vi "NML Data Acquisition-old.vi"() -> ()   [LabVIEW 2019]
doc: "This VI is designed to scan data each time the the trigger channel changes by an amount ∆ trigger. The first data column is converted to tesla using the magnet ID (or 'None' for volts).\nScott Hannahs, NHMFL - FSU, Mar 1996"
panel:
  in  "Configure":bool
  in  "Show help":bool
  in  "Display?":bool[](array[boolean])=[FALSE, FALSE, FALSE, FALSE, FALSE, FALSE, FALSE, FALSE, FALSE, FALSE, FALSE, FALSE, FALSE, FALSE, FALSE]
  out "# of columns":i32
  out "Index":i32
  out "Data Array":dbl[][](array[numeric]) format="%.2f"
  in  "Print":bool
  out "Data Record":string
  in  "Column Headings":string[](array[string])=["Field", "Voltage1", "Voltage2", "Temp", "Timestamp", "", "", "", "", "", "", "", "", "", ""]
  in  "Scale Factors":dbl[](array[numeric])=[1.0, 1.0, 1.0, 1.0, 1.0, 1.0, 1.0, 1.0, 1.0, 1.0, 1.0, 1.0, 1.0, 1.0, 1.0, 1.0, 1.0, 1.0, 1.0] format="%.3e"
  in  "Magnet ID":i32(ring) items=["None"]
  in  "Comments":string="This data's for you!\n"
  in  "Monopolar\n\n\n\nBipolar":bool
  in  "Points Averaged":i32=128 min=1 max=32000 step=1
  out "Mode Indicator":string="Standby"
  in  "User Name":string="Conan The Scientist"
  in  "File Name":string="Test"
  in  "TEST\nGPIB":bool
  in  "New/Stop":bool
  in  "X-Axis":i32(ring)=1 items=["Point #", "Field", "Voltage1", "Voltage2", "Temp", "Timestamp", "", "", "", "", "", "", "", "", "", ""]
  in  "Pause":bool=TRUE
  out "Data Plot":cluster{dbl[], dbl[]}[](graph)
  in  "CHANNEL & RANGE SELECTOR":T1 {"0" scale=0.0..4.0; "7" scale=0.0..4.0; "6" scale=0.0..4.0; "5" scale=0.0..4.0; "4" scale=0.0..4.0; "3" scale=0.0..4.0; "2" scale=0.0..4.0; "1" scale=0.0..4.0}
  in  "Æ Trigger":dbl=0.025 min=0.0 format="%.3f"
  in  "Trigger Column":i32(ring)=1 items=["Time", "Field", "Voltage1", "Voltage2", "Temp", "Timestamp", "", "", "", "", "", "", "", "", "", ""]
  # "Run"
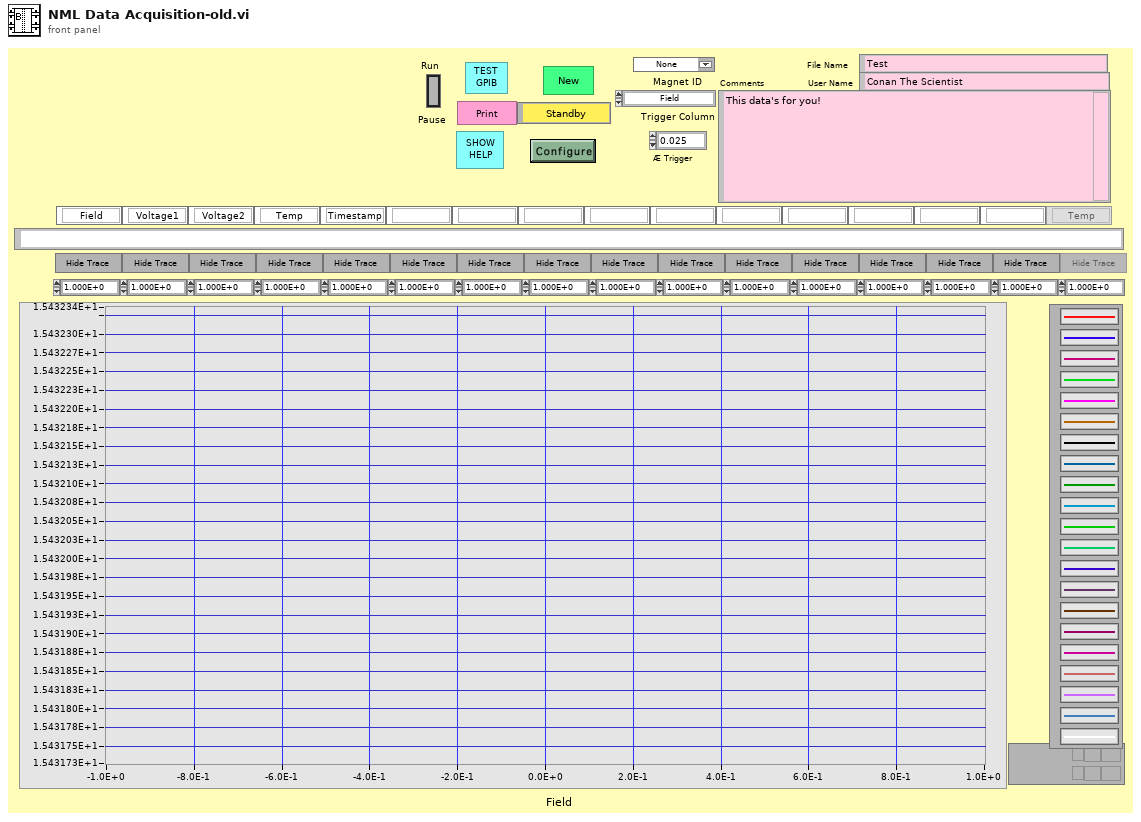
[diagram p1: front panel]
types:
  T1 = cluster{"0":i16, "1":i16, "2":i16, "3":i16, "4":i16, "5":i16, "6":i16, "7":i16}
  T2 = cluster{"Current Scale Factor kA/V":dbl, "I->B":dbl[], "B->I":dbl[]}
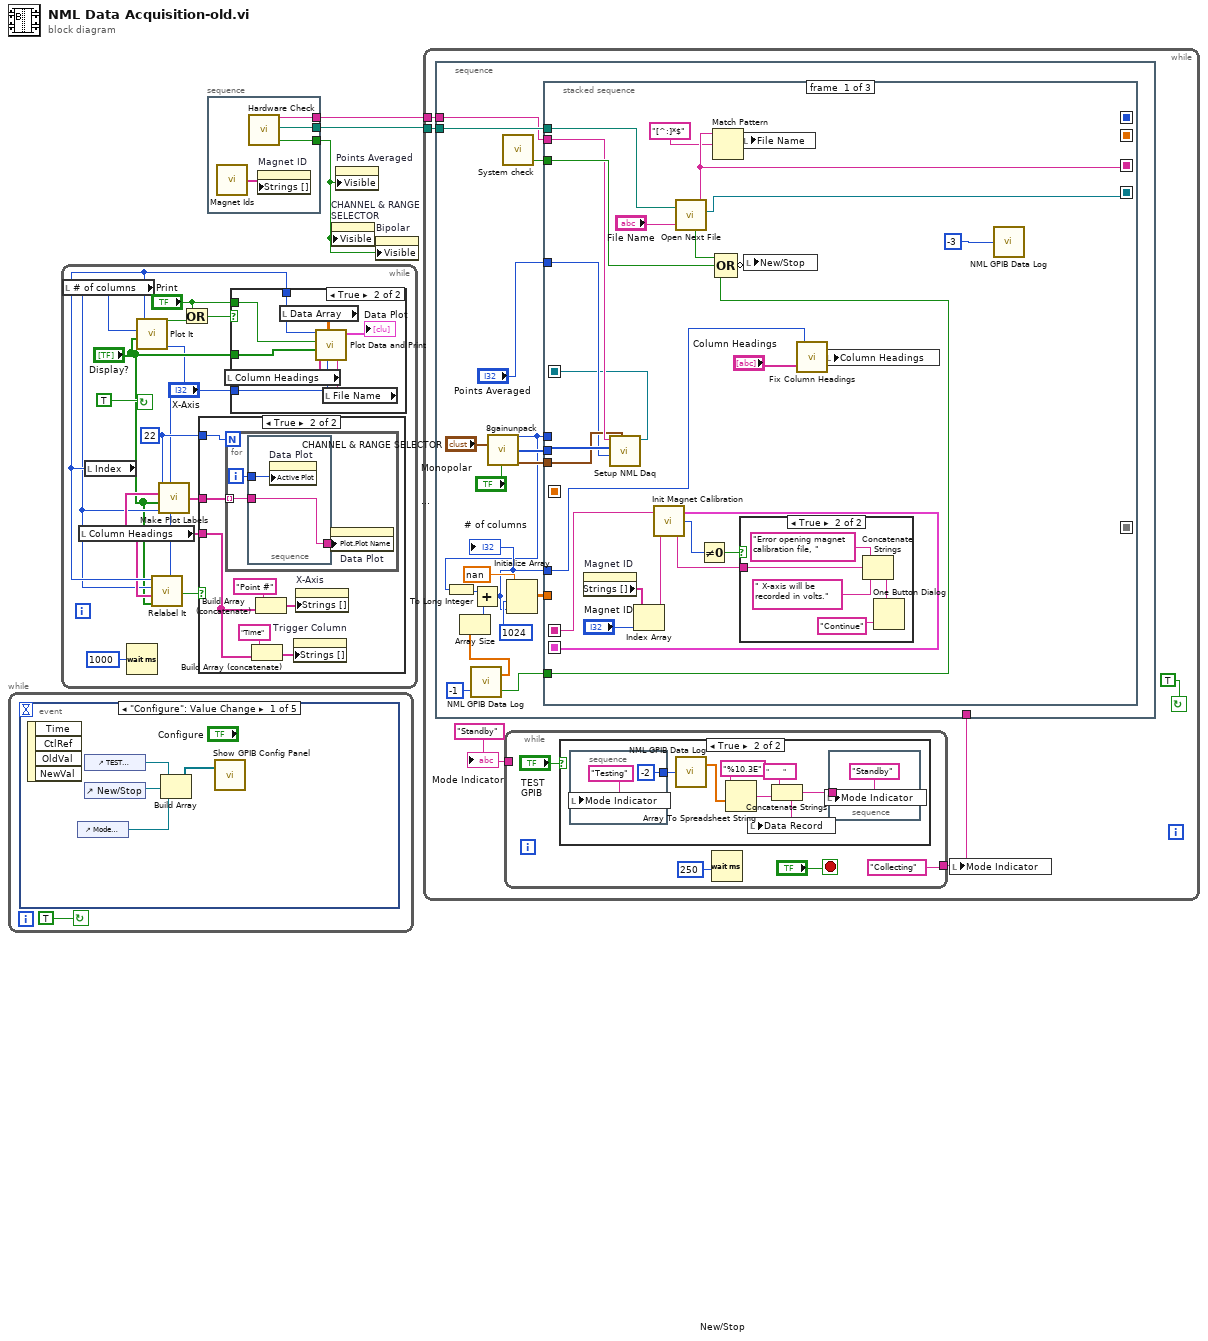
[diagram p0: block diagram]
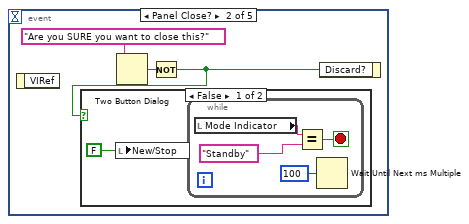
[diagram p2: hidden frame]
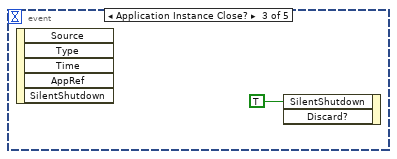
[diagram p4: hidden frame]
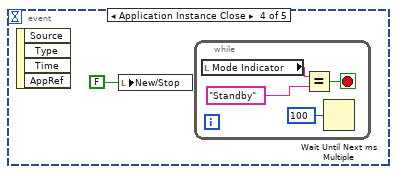
[diagram p5: hidden frame]
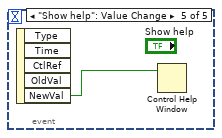
[diagram p6: hidden frame]
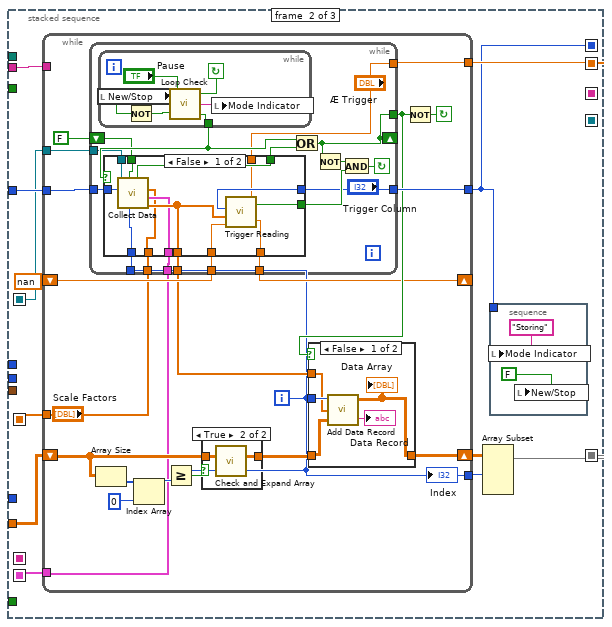
[diagram p9: hidden frame]
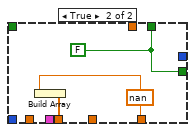
[diagram p10: hidden frame]
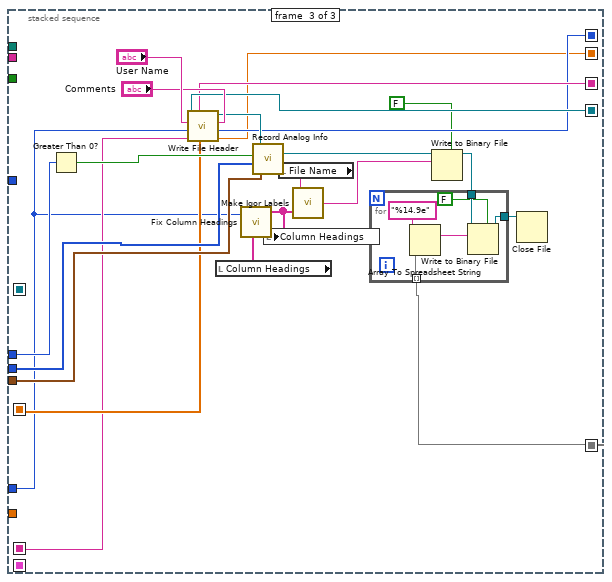
[diagram p13: hidden frame]
diagram:
  n1 = while {
    stop <- TRUE continue-if-true
    n2 = event shown="[0] \"Configure\": Value Change" {
      selector: _ -> [_ _ _ _ _]
      dyn-events: _ -> [_ _ _ _ _]
      timeout: _ -> [_ _ _ _ _]
      event "Configure": Value Change {
        n3 = event-data() -> ()  [unwired: 1 in, 4 out]
        n4 = control-ref of="Mode Indicator"() -> (w5:refnum<vi>)
        n5 = control-ref of="TEST\nGPIB"() -> (w7:refnum<vi>)
        n6 = control-ref of="New/Stop"() -> (w6:refnum<vi>)
        n7 = Build Array(w7, w6, w5) -> (w8:refnum<vi>[])
        n8 = call "Show GPIB Config Panel.vi"("Array"=w8) -> ()  [unwired: 1 in, 1 out]
      }
      event Panel Close? {
        n9 = event-data() -> ()  [unwired: 1 in, 1 out]
        n10 = Two Button Dialog(message="Are you SURE you want to close this?") -> (T button?=w10:bool)  [unwired: 2 in]
        n11 = Not(x=w10) -> (.not. x?=w9:bool)
        n12 = case shown="False" w9 {
          frame False {
            n13 = local write "New/Stop"(FALSE ("New/Stop")) -> ()
            n14 = while {
              stop <- w15 stop-if-true
              n15 = local read "Mode Indicator"() -> (w16:string)
              n16 = Equal?(x=w16, y="Standby") -> (x = y?=w15:bool)
              n17 = Wait Until Next ms Multiple(millisecond multiple=u32 100) -> ()  [unwired: 1 out]
            }
          }
          frame True {
          }
        }
        n18 = event-data("Discard?"=w9) -> ()  [unwired: 1 in, 1 out]
      }
      event Application Instance Close? {
        n19 = event-data() -> ()  [unwired: 1 in, 5 out]
        n20 = event-data("SilentShutdown"=TRUE) -> ()  [unwired: 2 in, 1 out]
      }
      event Application Instance Close {
        n21 = event-data() -> ()  [unwired: 1 in, 4 out]
        n22 = local write "New/Stop"(FALSE ("New/Stop")) -> ()
        n23 = while {
          stop <- w21 stop-if-true
          n24 = local read "Mode Indicator"() -> (w22:string)
          n25 = Equal?(x=w22, y="Standby") -> (x = y?=w21:bool)
          n26 = Wait Until Next ms Multiple(millisecond multiple=u32 100) -> ()  [unwired: 1 out]
        }
      }
      event "Show help": Value Change {
        n27 = event-data() -> ("NewVal"=w23:bool)  [unwired: 1 in, 4 out]
        n28 = Control Help Window(1:w23) -> ()  [unwired: 1 in]
      }
    }
  }
  n29 = while {
    stop <- TRUE continue-if-true
    w28 = 22
    n30 = local read "# of columns"() -> (w26:i32)
    n31 = local read "Column Headings"() -> (w27:string[])
    n32 = local read "Index"() -> (w30:i32)
    n33 = Wait (ms)(milliseconds to wait=u32 1000) -> ()  [unwired: 1 out]
    n34 = call "Plot It.vi"("X-Axis"="X-Axis", "Display?"="Display?", "# of columns"=w26, "Index"=w30) -> (0:w32:bool)
    n35 = call "Relabel It.vi"("Index"=w30, "# of columns"=w26, "Column Headings"=w27, "Display?"="Display?", "X-Axis"="X-Axis") -> (5:w34:bool)
    n36 = call "Make Plot Labels.vi"("Plot Size"=w28, "Column Headings"=w27, "Display?"="Display?", "# of columns"=w26, "X-axis"="X-Axis") -> ("Plot Names"=w29:string[])
    n37 = Or(x="Print", y=w32) -> (x .or. y?=w33:bool)
    n38 = case shown="True" w34 {
      tunnel: w27 -> [_ w37]
      tunnel: w28 -> [_ w39]
      tunnel: w29 -> [_ w38]
      frame False {
      }
      frame True {
        n39 = for {
          N: w39 -> [_]
          tunnel: w38 -> [w44] mode=indexing
          i -> [w46]
          n40 = stacked-sequence {
            tunnel: w46 -> [w48]
            tunnel: [w47] -> w45
            tunnel: w44 -> [w47]
            frame #0 {
              n41 = property on="Data Plot" class="XYGraph (strict)"("Active Plot"=w48) -> ()  [unwired: 2 in, 2 out]
            }
          }
          n42 = property on="Data Plot" class="XYGraph (strict)"("Plot.Plot Name"=w45) -> ()  [unwired: 2 in, 2 out]
        }
        n43 = Build Array (concatenate)("Time", w37) -> (w43:string[])
        n44 = Build Array (concatenate)("Point #", w37) -> (w41:string[])
        n45 = property on="Trigger Column" class="Ring (strict)"("Strings []"=w43) -> ()  [unwired: 2 in, 2 out]
        n46 = property on="X-Axis" class="Ring (strict)"("Strings []"=w41) -> ()  [unwired: 2 in, 2 out]
      }
    }
    n47 = case shown="True" w33 {
      tunnel: "Display?" -> [_ w56]
      tunnel: w30 -> [_ w55]
      tunnel: "X-Axis" -> [_ w50]
      tunnel: "Print" -> [_ w49]
      frame False {
      }
      frame True {
        n48 = local read "Column Headings"() -> (w51:string[])
        n49 = local read "Data Array"() -> (w52:dbl[][])
        n50 = local read "File Name"() -> (w54:string)
        n51 = call "Plot Data and Print.vi"("File:"=w54, "x axis column"=w50, "Data"=w52, "Col heading"=w51, "Display/hide"=w56, "Print"=w49, "Index"=w55) -> ("Data Plot"=→"Data Plot":cluster{dbl[], dbl[]}[])  [unwired: 2 in]
      }
    }
  }
  n52 = stacked-sequence {
    tunnel: [w59] -> w1
    tunnel: [w58] -> w2
    tunnel: [w57] -> w3
    frame #0 {
      n53 = call "Magnet Ids.vi"() -> ("Magnet IDs"=w60:string[])
      n54 = call "Hardware Check.vi"() -> ("Data Acq Device"=w57:string, "Data Directory Path"=w59:path, "Has A/D board"=w58:bool)  [unwired: 1 in]
      n55 = property on="Magnet ID" class="Ring (strict)"("Strings []"=w60) -> ()  [unwired: 2 in, 2 out]
    }
  }
  n56 = property on="CHANNEL & RANGE SELECTOR" class="Clust (strict)"("Visible"=w2) -> ()  [unwired: 2 in, 2 out]
  n57 = property on="Points Averaged" class="DigNum (strict)"("Visible"=w2) -> ()  [unwired: 2 in, 2 out]
  n58 = property on="Bipolar" class="Bool (strict)"("Visible"=w2) -> ()  [unwired: 2 in, 2 out]
  n59 = while {
    tunnel: w3 -> [w63]
    tunnel: w1 -> [w64]
    stop <- TRUE continue-if-true
    w62 = "Standby"
    n60 = while {
      tunnel: ["Collecting"] -> w61
      tunnel: w62 -> [_]
      stop <- "New/Stop" stop-if-true
      n61 = case shown="True" "TEST\nGPIB" {
        frame False {
        }
        frame True {
          n62 = stacked-sequence {
            tunnel: [-2] -> w71
            frame #0 {
              n63 = local write "Mode Indicator"("Testing") -> ()
            }
          }
          n64 = call "NML GPIB Data Log.vi"("Point #"=w71) -> ("GPIB Data"=w70:dbl[])  [unwired: 1 out]
          n65 = Array To Spreadsheet String(array=w70, 3:"%10.3E") -> (spreadsheet string=w73:string)  [unwired: 1 in]
          n66 = Concatenate Strings("       ", w73) -> (w74:string)
          n67 = local write "Data Record"(w74) -> ()
          n68 = stacked-sequence {
            tunnel: w74 -> [_]
            frame #0 {
              n69 = local write "Mode Indicator"("Standby") -> ()
            }
          }
        }
      }
      n70 = Wait (ms)(milliseconds to wait=u32 250) -> ()  [unwired: 1 out]
    }
    n71 = stacked-sequence {
      tunnel: w64 -> [w89]
      tunnel: w63 -> [w88]
      tunnel: w61 -> [_]
      frame #0 {
        n72 = call "NML GPIB Data Log.vi"("Point #"=-1) -> ("GPIB Data"=w80:dbl[], "Stop"=w81:bool)
        n73 = Array Size(array=w80) -> (size(s)=w94:i32)
        n74 = call "8gainunpack.vi"("GAIN & CHANNEL SELECTOR"="CHANNEL & RANGE SELECTOR", "Monopolar"="Monopolar\n\n\n\nBipolar") -> ("Number of channels"=w82:i32, "channels (0)"=w93:i32[], "Input Limits"=w96:cluster{"High Limit":dbl, "Low Limit":dbl}[])
        n75 = To Long Integer(number=w82) -> (32bit integer=w95:i32)
        n76 = Add(x=w95, y=w94) -> (x+y=w85:i32)
        "# of columns" <- w85
        n77 = call "System check.vi"() -> ("Abort"=w84:bool)  [unwired: 3 in]
        n78 = Initialize Array(nan, 1024, w85) -> (w92:dbl[][])
        n79 = stacked-sequence "file Name" {
          seq-local: [_ w130 _] -> [_ _ w214]
          seq-local: [_ w136 _] -> [_ _ w230]
          seq-local: [_ w139 _] -> [_ _ w213]
          seq-local: [w104 _ _] -> [_ _ w216]
          seq-local: [w117 _ _] -> [_ w138 _]
          seq-local: [w122 _ _] -> [_ _ w217]
          seq-local: [w119 _ _] -> [_ _ w215]
          seq-local: [_ w134 _] -> [_ _ w220]
          seq-local: [w98 _ _] -> [_ w128 _]
          tunnel: w92 -> [_ w131 _]
          tunnel: w88 -> [w102 w137 _]
          tunnel: w96 -> [w101 _ w231]
          tunnel: w93 -> [w103 _ w232]
          tunnel: w82 -> [_ _ w212]
          tunnel: w85 -> [w99 _ w211]
          tunnel: w89 -> [w110 _ _]
          tunnel: w84 -> [w108 _ _]
          tunnel: w81 -> [w107 _ _]
          tunnel: "Points Averaged" -> [w100 w129 _]
          frame #0 {
            n80 = property on="Magnet ID" class="Ring (strict)"() -> ("Strings []"=w106:string[])  [unwired: 2 in, 2 out]
            n81 = call "Setup NML Daq.vi"("Input Limits"=w101, "number of samples per channel"=w100, "channels (0)"=w103, "Data Acq Device"=w102) -> ("task out"=w98:refnum<k21>)  [unwired: 6 in, 1 out]
            n82 = Index Array(array=w106, index="Magnet ID") -> (element=w104:string)
            n83 = call "Init Magnet Calibration.vi"("Magnet Id"=w104) -> ("Calibration"=w117:T2, "Error Code"=w120:i32, "Error message"=w111:string)
            n84 = call "Open Next File.vi"("Input File Pattern"="File Name", "Dir Path"=w110) -> ("File Ref Num"=w122:refnum<file>, "Output File Name"=w119:string, "Stop"=w109:bool)  [unwired: 1 in, 1 out]
            n85 = Not Equal To 0?(x=w120) -> (x != 0?=w121:bool)
            n86 = Match Pattern(string=w119, regular expression="[^:]*$") -> (match substring=w115:string)  [unwired: 1 in, 3 out]
            n87 = Compound Arithmetic op=OR(w109, w108, w107) -> (invert w112:bool)
            n88 = case shown="True" w121 {
              tunnel: w111 -> [_ w123]
              frame False {
              }
              frame True {
                n89 = Concatenate Strings("Error opening magnet calibration file, ", w123, " X-axis will be recorded in volts.") -> (w125:string)
                n90 = One Button Dialog(message=w125, button name ("OK")="Continue") -> ()  [unwired: 1 out]
              }
            }
            n91 = local write "File Name"(w115) -> ()
            n92 = local write "New/Stop"(w112) -> ()
            n93 = call "Fix Column Headings.vi"("Column Headings"="Column Headings", "# Cols"=w99) -> ("Column Headings"=w113:string[])
            n94 = local write "Column Headings"(w113) -> ()
            n95 = call "NML GPIB Data Log.vi"("Point #"=-3) -> ()  [unwired: 2 out]
          }
          frame #1 {
            n96 = while {
              tunnel: ["Scale Factors"] -> w134
              tunnel: w138 -> [w146]
              tunnel: [w158] -> w139
              tunnel: w137 -> [_]
              tunnel: [w142] -> w132
              tunnel: [w151] -> w130
              shift-left: nan -> [w148]
              shift-right: [w149] -> _
              shift-left: w131 -> [w154]
              shift-right: [w159] -> w133
              tunnel: w129 -> [w141]
              tunnel: w128 -> [w140]
              i -> [w142]
              stop <- w144 continue-if-true
              n97 = while {
                shift-left: FALSE -> [w161]
                shift-right: [w160] -> _
                tunnel: w140 -> [w173]
                tunnel: [w160] -> w150
                tunnel: ["Æ Trigger"] -> w158
                tunnel: w141 -> [w168]
                tunnel: ["Trigger Column"] -> w151
                tunnel: w148 -> [w170]
                tunnel: [w169] -> w149
                tunnel: w142 -> [w167]
                tunnel: [w166] -> w147
                tunnel: w146 -> [w165]
                tunnel: "Scale Factors" -> [w164]
                stop <- w175 continue-if-true
                n98 = while {
                  tunnel: [w180] -> w174
                  stop <- w181 continue-if-true
                  n99 = local read "New/Stop"() -> (w178:bool)
                  n100 = Not(x=w178) -> (.not. x?=w179:bool)
                  n101 = call "Loop Check.vi"("Pause"="Pause", "Stop"=w179) -> ("Pause"=w181:bool, "State"=w177:string, "ABORT"=w180:bool)
                  n102 = local write "Mode Indicator"(w177) -> ()
                }
                n103 = case shown="False" w174 {
                  tunnel: "Æ Trigger" -> [w185 _]
                  tunnel: w161 -> [w186 _]
                  tunnel: [w187 w198] -> w163
                  tunnel: w164 -> [w183 _]
                  tunnel: w165 -> [w188 _]
                  tunnel: [w189 w196] -> w166
                  tunnel: w167 -> [w190 _]
                  tunnel: w168 -> [w191 _]
                  tunnel: [w184 w197] -> w169
                  tunnel: w170 -> [w192 _]
                  tunnel: "Trigger Column" -> [w193 _]
                  tunnel: [w194 w198] -> w172
                  tunnel: w173 -> [w195 _]
                  frame False {
                    n104 = call "Collect Data.vi"("Calibration"=w188, "Scaling Factors"=w183, "Point Number"=w190, "stop"=w186, "Number to Average"=w191, "task"=w195) -> ("Output Data"=w189:dbl[], "Stop"=w187:bool)  [unwired: 3 in]
                    n105 = call "Trigger Reading.vi"("Old Trigger Value"=w192, "Current Values"=w189, "Trigger Column"=w193, "Æ Trigger Value"=w185) -> ("New Trigger Value"=w184:dbl, "Wait"=w194:bool)
                  }
                  frame True {
                    w198 = FALSE
                    w197 = nan
                    n106 = Build Array(w197) -> (w196:dbl[])
                  }
                }
                n107 = Or(x=w174, y=w163) -> (x .or. y?=w160:bool)
                n108 = Not(x=w160) -> (.not. x?=w176:bool)
                n109 = And(x=w176, y=w172) -> (x .and. y?=w175:bool)
              }
              n110 = Array Size(array=w154) -> (size(s)=w152:i32[])
              n111 = Index Array(array=w152, index=0) -> (element=w157:i32)
              n112 = Greater Or Equal?(x=w142, y=w157) -> (x >= y?=w155:bool)
              n113 = case shown="True" w155 {
                tunnel: [w205 w206] -> w153
                tunnel: w154 -> [w205 w207]
                frame False {
                }
                frame True {
                  n114 = call "Check and Expand Array.vi"(1:w207) -> (0:w206:dbl[][])
                }
              }
              n115 = case shown="False" w150 {
                tunnel: w147 -> [w200 _]
                tunnel: [w199 w204] -> w159
                tunnel: w142 -> [w203 _]
                tunnel: w153 -> [w202 w204]
                frame False {
                  n116 = call "Add Data Record.vi"("Data In"=w202, "Data to update"=w200, "Index"=w203) -> ("Data Display"=→"Data Record":string, "Data Out"=w199:dbl[][])  [unwired: 1 in]
                  "Data Array" <- w199
                }
                frame True {
                }
              }
              n117 = Not(x=w150) -> (.not. x?=w144:bool)
              "Index" <- w142
            }
            n118 = Array Subset(array=w133, length (row)=w132) -> (w136:dbl[][])  [unwired: 3 in]
            n119 = stacked-sequence {
              tunnel: w130 -> [_]
              frame #0 {
                n120 = local write "Mode Indicator"("Storing") -> ()
                n121 = local write "New/Stop"(FALSE) -> ()
              }
            }
          }
          frame #2 {
            n122 = Greater Than 0?(x=w212) -> (x > 0?=w229:bool)
            n123 = call "Write File Header.vi"("Æ Trigger"=w213, "Trigger Column"=w214, "Comments"="Comments", "Scale Factors"=w220, "Output File Name"=w215, "Magnet Id"=w216, "# Cols"=w211, "User Name"="User Name", "File Ref Num 2"=w217) -> ("File Ref Num"=w218:refnum<file>)
            n124 = local read "Column Headings"() -> (w228:string[])
            n125 = call "Fix Column Headings.vi"("Column Headings"=w228, "# Cols"=w211) -> ("Column Headings"=w227:string[])
            n126 = call "Record Analog Info.vi"("input limits (no change)"=w231, "channels (0)"=w232, "Boolean"=w229, "File Ref Num 2"=w218) -> ("File Ref Num"=w222:refnum<file>)
            n127 = local write "Column Headings"(w227) -> ()
            n128 = local read "File Name"() -> (w225:string)
            n129 = call "Make Igor Labels.vi"("Column Names"=w227, "File Name"=w225) -> ("Igor Column Headings"=w226:string)
            n130 = Write to Binary File(file (use dialog)=w222, data=w226, 5:FALSE ("prepend array or string size? (T)")) -> (refnum out=w223:refnum<file>)  [unwired: 3 in, 2 out]
            n131 = for {
              tunnel: w230 -> [w237] mode=indexing
              tunnel: w223 -> [w234]
              tunnel: [w235] -> w224
              n132 = Array To Spreadsheet String(array=w237, 3:"%14.9e") -> (spreadsheet string=w236:string)  [unwired: 1 in]
              n133 = Write to Binary File(file (use dialog)=w234, data=w236, 5:FALSE ("prepend array or string size? (T)")) -> (refnum out=w235:refnum<file>)  [unwired: 3 in, 2 out]
            }
            n134 = Close File(refnum=w224) -> ()  [unwired: 1 in, 2 out]
          }
        }
      }
    }
    n135 = local write "Mode Indicator"(w61) -> ()
    "Mode Indicator" <- w62
  }
